vi "Make Y=0 waveform.vi"(8 "Error In (no Error) In":errorcluster, 11 "Signal In":waveform(dbl)) -> (0 "Error Out":errorcluster, 3 "Signal Out":waveform(dbl))   [LabVIEW 2018, in "Waveform Control.xctl"]
doc: "Generates a waveform that is all 0, but with same time information as the input array and returns both as an array of waveforms. Used to generate the plots for the graphical waveform display"
uses:
  Waveform Control.xctl
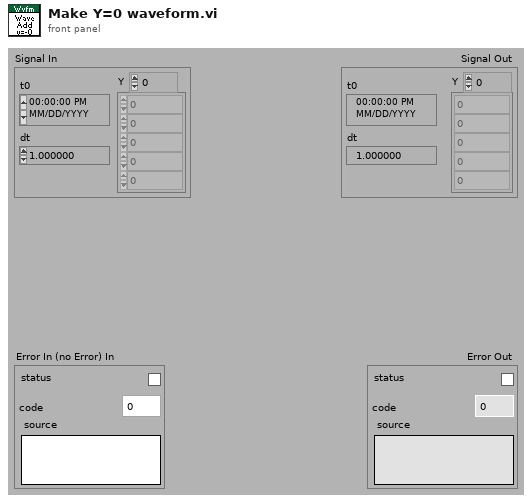
[diagram p1: front panel]
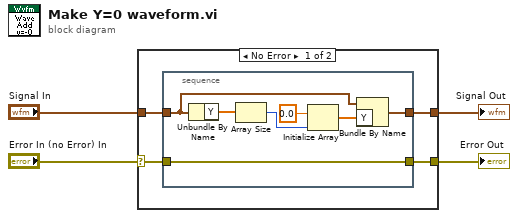
[diagram p0: block diagram]
diagram:
  n1 = case shown="No Error" "Error In (no Error) In" {
    selector: "Error In (no Error) In" -> [w5 w16]
    tunnel: [w8 _] -> w4
    tunnel: "Signal In" -> [w7 _]
    tunnel: [w6 w16] -> w2
    frame No Error {
      n2 = stacked-sequence {
        tunnel: [w15] -> w8
        tunnel: w7 -> [w13]
        tunnel: [w9] -> w6
        tunnel: w5 -> [w9]
        frame #0 {
          n3 = Unbundle By Name(w13) -> ("Y"=w10:dbl[])
          n4 = Array Size(array=w10) -> (size(s)=w11:i32)
          n5 = Initialize Array(0.0 ("element"), w11) -> (w14:dbl[])
          n6 = Bundle By Name(cluster=w13, "Y"=w14) -> (w15:waveform(dbl))
        }
      }
    }
    frame Error {
    }
  }
  "Signal Out" <- w4
  "Error Out" <- w2
